vi "P3060_DMA读U8数据.vi"(8 "错误输入":errorcluster caption="错误输入（无错误）", 9 "数据长度":u32, 10 "偏移地址":u32, 11 "句柄输入":i32) -> (0 "错误输出":errorcluster, 1 "读U8数据":u8[](array[numeric]), 2 "返回值":i32, 3 "句柄输出":i32)   [LabVIEW 2010]
doc: "发送异步通道数据"
uses:
  dll/P3060.dll
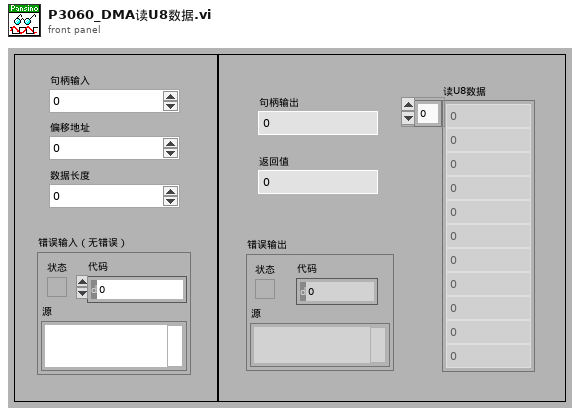
[diagram p1: front panel]
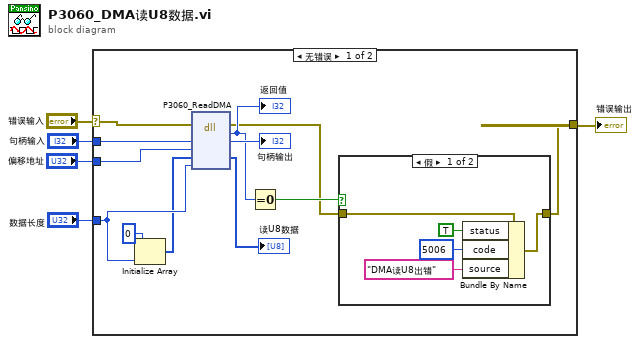
[diagram p0: block diagram]
diagram:
  n1 = case shown="无错误" "错误输入" {
    selector: "错误输入" -> [w17 w24]
    tunnel: [w11 w24] -> w3
    tunnel: "数据长度" -> [w8 _]
    tunnel: "句柄输入" -> [w15 _]
    tunnel: "偏移地址" -> [w10 _]
    frame No Error {
      n2 = Initialize Array(u8 0, w8) -> (w7:u8[])
      n3 = dll-call lib="D:/driver/trunk/Drivers/P3060/P3060API/P3060APILV/Labview/P3060/_SubVI/dll/P3060.dll" fn="P3060_ReadDMA"(error in=w17, "hDev"=w15, "Offset"=w10, "pBuffer"=w7, "lengthToWrite"=w8) -> (error out=w12:errorcluster, "return"=w14:i32, "hDev"=→"句柄输出":i32, "pBuffer"=→"读U8数据":u8[])  [unwired: 4 in, 1 out]
      "返回值" <- w14
      n4 = Equal To 0?(x=w14) -> (x = 0?=w13:bool)
      n5 = case shown="假" w13 {
        tunnel: [w21 w23] -> w11
        tunnel: w12 -> [w22 w23]
        frame False {
          n6 = Bundle By Name(cluster=w22, "status"=TRUE, "code"=5006, "source"="DMA读U8出错") -> (w21:errorcluster)
        }
        frame True {
        }
      }
    }
    frame Error {
    }
  }
  "错误输出" <- w3
